vi "BuildJoystickGraph.vi"(1 "YAxis":dbl, 2 "XAxis":dbl) -> (0 "Left Joystick":cluster{dbl[], dbl[]}(graph))   [LabVIEW 2012]
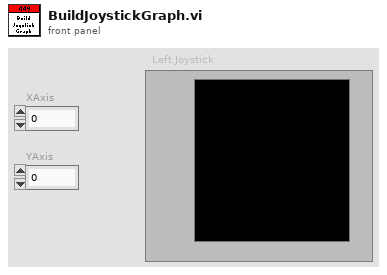
[diagram p1: front panel]
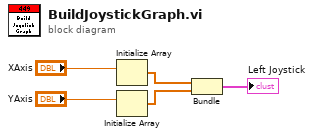
[diagram p0: block diagram]
diagram:
  n1 = Initialize Array("XAxis") -> (w5:dbl[])  [unwired: 1 in]
  n2 = Initialize Array("YAxis") -> (w4:dbl[])  [unwired: 1 in]
  n3 = Bundle(w5, w4) -> (→"Left Joystick":cluster{dbl[], dbl[]})  [unwired: 1 in]
